vi "Read Sample from Container.vi"(8 "error in (no error)":errorcluster, 10 "Container":T1, 11 "Syringe Line in":refnum<class "Syringe Line.lvclass">) -> (0 "error out":errorcluster, 2 "Sample":refnum<class "Sample.lvclass">, 3 "Syringe Line out":refnum<class "Syringe Line.lvclass">)   [LabVIEW 2015, in "cRIO-Carbondioxide.lvlib" / "CO2-Actor.lvlib" / "Syringe Line.lvclass"]
uses:
  Syringe Line.lvclass
  Controls/Sample Transfer Container Enumerator.ctl
  subs/Sample/Sample.lvclass
  CO2 Actor/CO2 Actor.lvclass
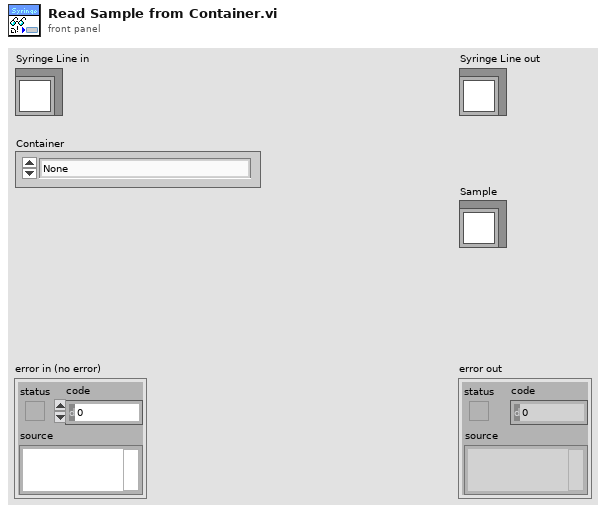
[diagram p1: front panel]
types:
  T1 = typedef "Sample Transfer Container Enumerator.ctl" = enum16{"None", "Sample 1", "Sample 2", "Sample 3", "Sample 4", "Sample 5", "Storage 01", "Storage 02", "Storage 03", "Storage 04", "Storage 05", "Storage 06", "Storage 07", "Storage 08", "Storage 09", "Storage 10", "Storage 11", "Storage 12", "Syringe", "Undefined"}
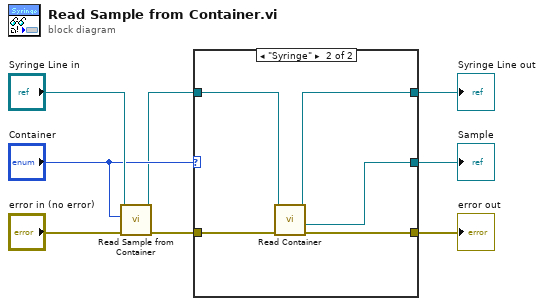
[diagram p0: block diagram]
diagram:
  n1 = call-parent "Read Sample from Container.vi"("error in (no error)"="error in (no error)", "Container"="Container", "CO2 Actor in"="Syringe Line in") -> ("error out"=w6:errorcluster, "CO2 Actor out"=w3:refnum<class "Syringe Line.lvclass">)  [unwired: 6 in, 1 out]
  n2 = case shown="\"Syringe\"" "Container" {
    tunnel: w6 -> [w9 w15]
    tunnel: [w10 w12] -> w4
    tunnel: w3 -> [w10 w13]
    tunnel: [w9 w14] -> w2
    tunnel: [_ w11] -> w1
    frame "None", Default {
    }
    frame "Syringe" {
      n3 = call "Read Container.vi"("error in (no error)"=w15, "Syringe Line in"=w13) -> ("error out"=w14:errorcluster, "Sample"=w11:refnum<class "Sample.lvclass">, "Syringe Line out"=w12:refnum<class "Syringe Line.lvclass">)  [unwired: 6 in, 1 out]
    }
  }
  "error out" <- w2
  "Syringe Line out" <- w4
  "Sample" <- w1
